vi "Export Origin - CV.vi"(8 "Error In":errorcluster, 9 "Workspace":path, 10 "Session properties":T4, 11 "CV measurement":T1={"Name"="", "Comment"="", "Time"=timestamp(0 s since 1904-01-01), "Folder"=path "", "CV properties"={"T"=0.0, "Vstart"=-0.5, "Vstop"=0.5, "Vpoints"=10.0, "Precision"=enum."Normal", "Test signal"=0.01, "Auto I range"=FALSE, "Test frequency"=100000.0, "I range"=-2.0, "V range"=10.0, "Log mapping"=FALSE, "Rel perm"=0.0, "Area"=0.0}, "GUID"=""} {"CV properties"."V range" items=["10mV"=0.01, "100mV"=0.1, "1V"=1.0, "10V"=10.0]; "CV properties"."I range" items=["100nA"=-7.0, "1µA"=-6.0, "10µA"=-5.0, "100µA"=-4.0, "1mA"=-3.0, "10mA"=-2.0]}) -> (0 "Error Out":errorcluster)   [LabVIEW 2019]
doc: "Handles export of a C-V measurement to an Origin project, displays a GUI window"
uses:
  <vilib>/Utility/sysdir.llb/System Directory Type.ctl
  Type defs/Session properties Type Def.ctl
  Type defs/CV properties Type Def.ctl
  Type defs/CV measurement Type Def.ctl
panel:
  in  "Comment":T3(array[ring])=[enum."Temperature"] caption="Parameters to be placed in comments"
  in  "Save and exit after export":bool
  in  "Export to current Origin instance":bool
  out "String":string
  in  "Path":path caption="Export file as:"
  in  "Export":bool
  in  "Cancel":bool
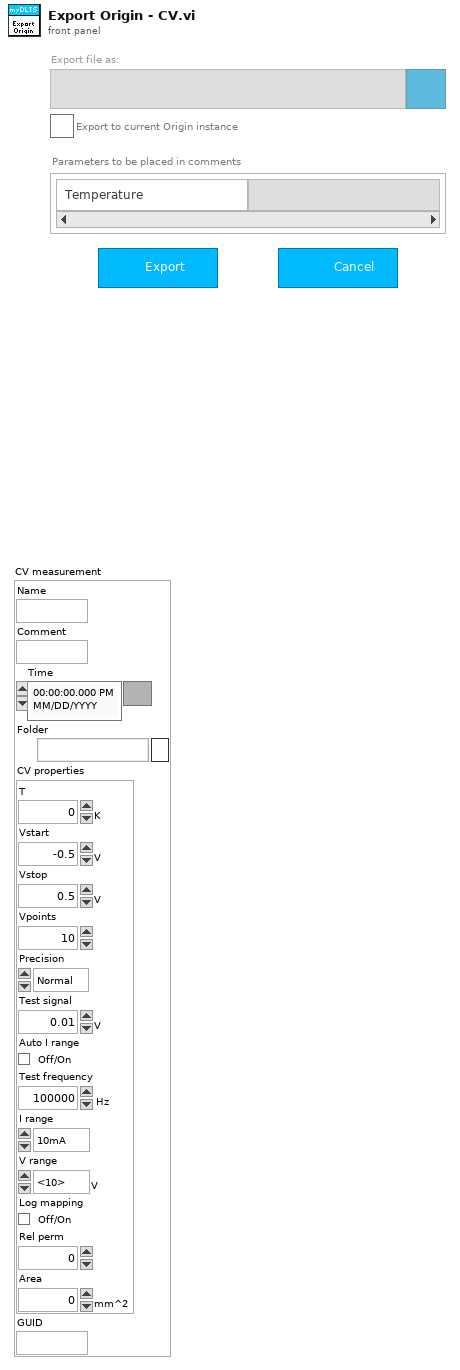
[diagram p1: front panel]
types:
  T1 = typedef "CV measurement Type Def.ctl" = cluster{"Name":string, "Comment":string, "Time":timestamp, "Folder":path, "CV properties":T2, "GUID":string}
  T2 = typedef "CV properties Type Def.ctl" = cluster{"T":dbl[unit], "Vstart":dbl[unit], "Vstop":dbl[unit], "Vpoints":dbl, "Precision":enum16{"Low (Fast)", "Normal", "High (Slow)"}, "Test signal":dbl[unit], "Auto I range":bool, "Test frequency":dbl[unit], "I range":dbl, "V range":dbl[unit], "Log mapping":bool, "Rel perm":dbl, "Area":dbl[unit]}
  T3 = enum16{"", "Temperature", "Test signal", "Test frequency", "Current range", "Voltage range"}[]
  T4 = typedef "Session properties Type Def.ctl" = cluster{"Session name":string, "Comment":string, "User":string, "Software version":dbl, "Created":timestamp, "Modified":timestamp, "Binary":bool, "GUID":string}
  T5 = enum32{"existing file", "new file", "new or existing file", "existing dir", "new dir", "new or existing dir", "existing file (use LLBs)", "new file (use LLBs)", "new or existing file (use LLBs)", "new or existing file or directory (use LLBs)", "existing dir (use LLBs)", "new dir (use LLBs)", "new or existing dir (use LLBs)", "existing file or dir", "new file or dir", "new or existing file or dir", "existing file or dir (use LLBs)", "new file or dir (use LLBs)"}
  T6 = enum8{"Enabled", "Disabled", "Disabled and Grayed Out"}
  T7 = typedef "System Directory Type.ctl" = i32
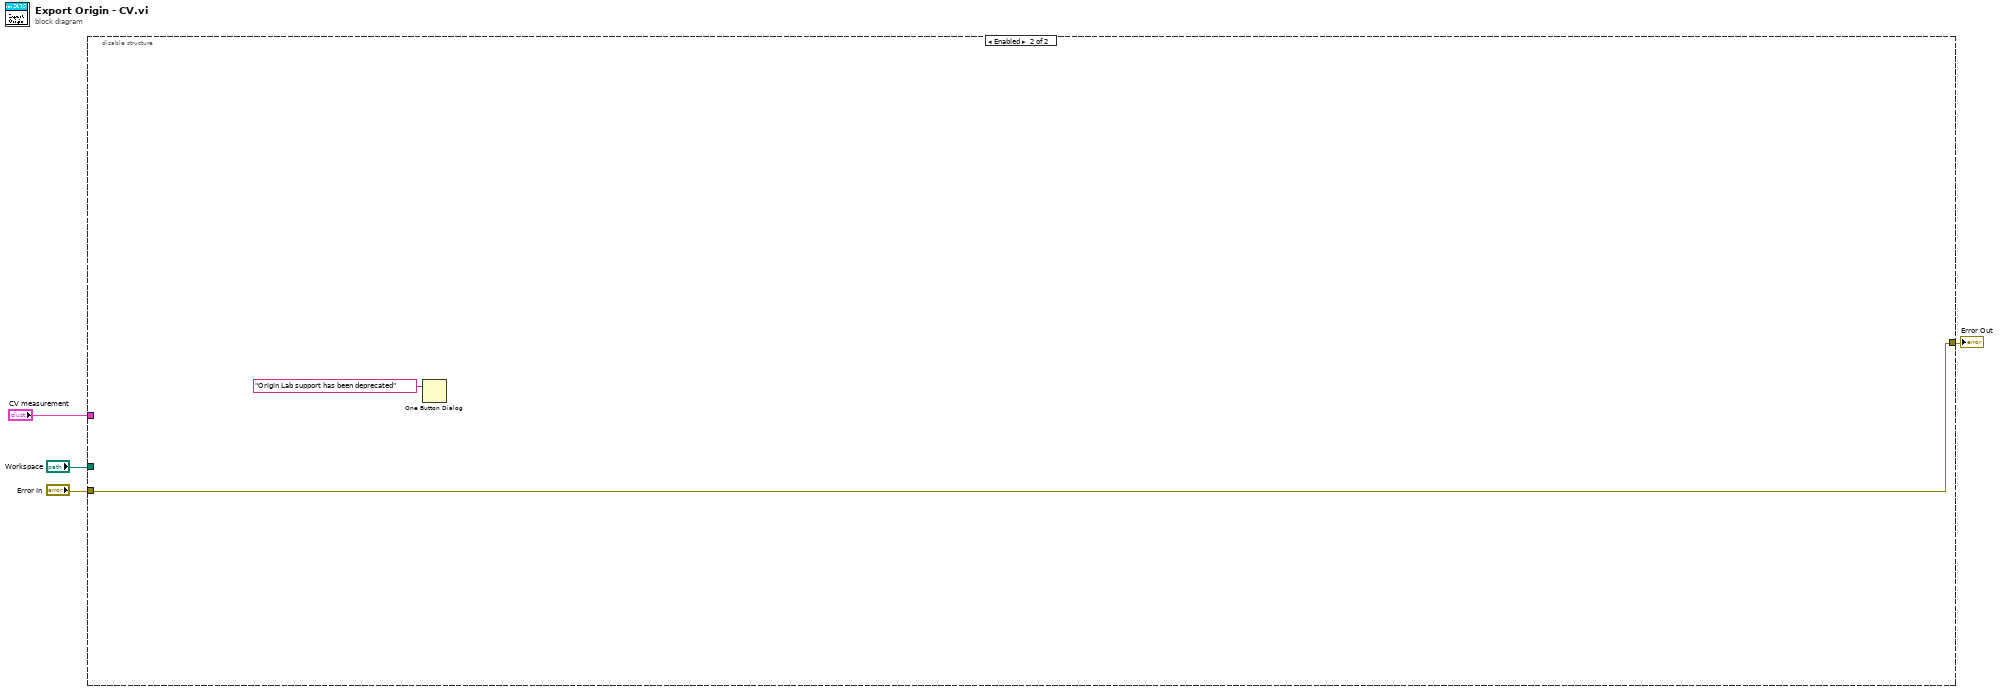
[diagram p0: block diagram]
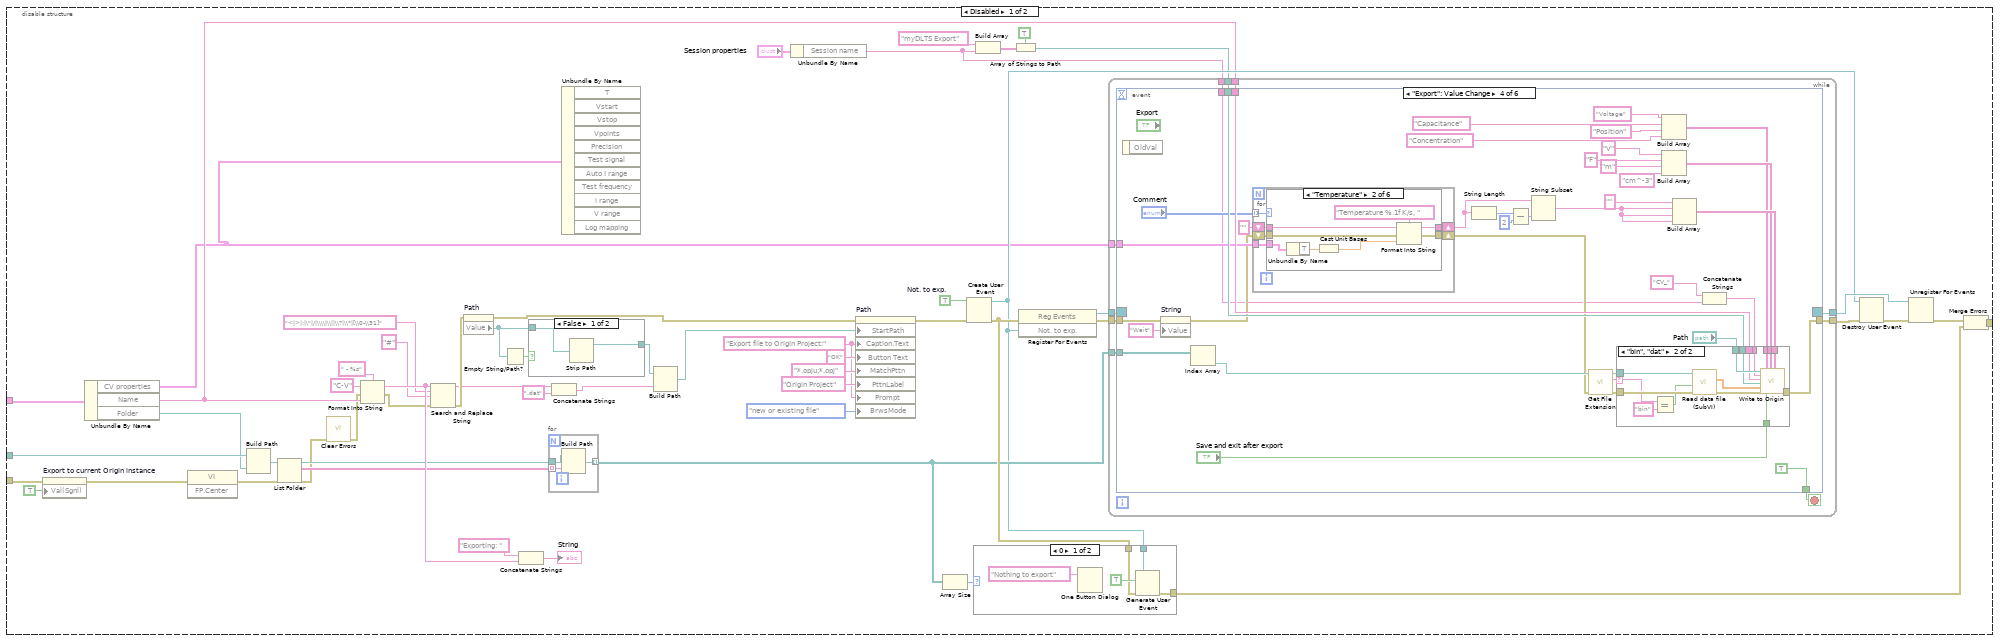
[diagram p2: hidden frame]
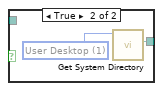
[diagram p3: hidden frame]
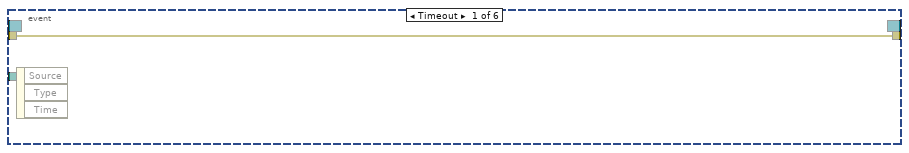
[diagram p5: hidden frame]
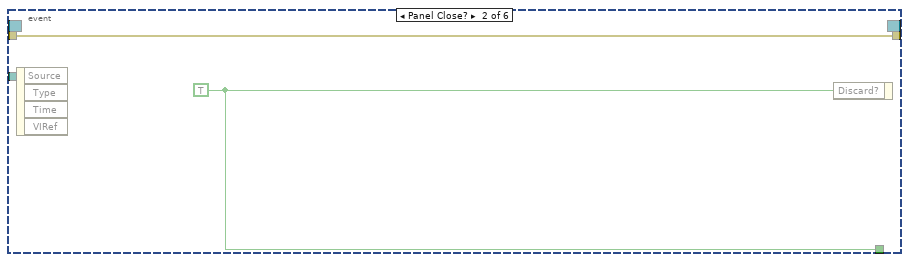
[diagram p6: hidden frame]
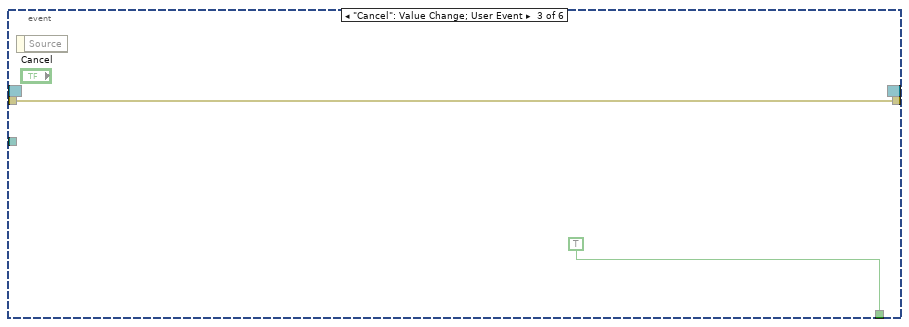
[diagram p7: hidden frame]
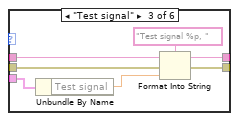
[diagram p9: hidden frame]
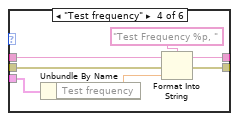
[diagram p10: hidden frame]
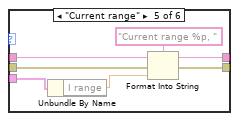
[diagram p11: hidden frame]
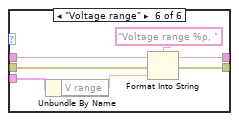
[diagram p12: hidden frame]
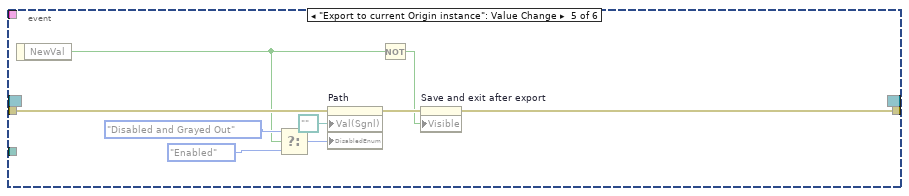
[diagram p14: hidden frame]
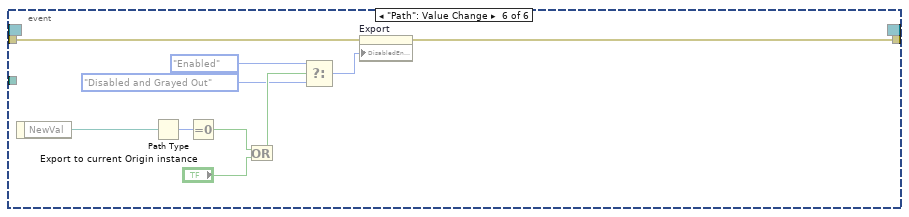
[diagram p15: hidden frame]
diagram:
  n1 = disable-structure shown="Enabled" {
    disable-tunnel: "Workspace" -> [w60 _]
    disable-tunnel: [w49 w207] -> w3
    disable-tunnel: "Error In" -> [w11 w207]
    disable-tunnel: "CV measurement" -> [w8 _]
    frame Disabled {
      w31 = "Export file to Origin Project:"
      w58 = TRUE  # Not. to exp.
      n2 = property on="Export to current Origin instance" class="Bool (strict)"(error in=w11, "Val(Sgnl)"=TRUE ("Value (Signaling)")) -> (error out=w10:errorcluster)  [unwired: 1 in, 1 out]
      n3 = Unbundle By Name(w8) -> ("CV properties"=w7:T2, "Name"=w18:string, "Folder"=w36:path)
      n4 = invoke class="VI" method="FP.Center"(error in=w10) -> (error out=w20:errorcluster)  [unwired: 2 in, 2 out]
      n5 = Build Path(base path=w60, name or relative path=w36) -> (appended path=w29:path)
      n6 = List Folder(path=w29, error in=w20) -> (path out=w28:path, filenames=w35:string[], error out=w24:errorcluster)  [unwired: 2 in, 1 out]
      n7 = call <vilib>:"Clear Errors.vi"("error in (no error)"=w24) -> ("error out"=w5:errorcluster)  [unwired: 5 in, 1 out]
      n8 = Format Into String(format string=" - %s", initial string="C-V", error in=w5, w18) -> (resulting string=w47:string, error out=w23:errorcluster)
      n9 = Search and Replace String(input string=w47, search string="<|>|:|\"|/|\\\\|\\||\\?|\\*|[\\0-\\31]", replace string="#" ("replace string (\"\")"), error in=w23) -> (result string=w22:string, error out=w25:errorcluster)  [unwired: 4 in, 2 out]
      n10 = property on="Path" class="Path"(error in=w25) -> (error out=w37:errorcluster, "Value"=w43:path)  [unwired: 1 in, 1 out]
      n11 = Empty String/Path?(string/path=w43) -> (empty?=w44:bool)
      n12 = Concatenate Strings("Exporting: " ("string"), w47) -> (→"String":string)
      n13 = case shown="False" w44 {
        tunnel: w43 -> [w65 _]
        tunnel: [w64 w66] -> w39
        frame False {
          n14 = Strip Path(path=w65) -> (stripped path=w64:path)  [unwired: 1 out]
        }
        frame True {
          w67 = T7 1 items=["User Home"=0, "User Desktop"=1, "User Documents"=2, "User Application Data"=3, "User Preferences"=4, "User Temporary"=5, "Public Documents"=6, "Public Application Data"=7, "Public Preferences"=8, "Public Cache"=13, "System Core Libraries"=9, "System Installed Libraries"=10, "Application Files"=11, "Boot Volume Root"=12] ("system directory type")
          n15 = call <vilib>:"Get System Directory.vi"("system directory type"=w67) -> ("system directory"=w66:path)  [unwired: 10 in]
        }
      }
      n16 = for {
        tunnel: w28 -> [w63]
        tunnel: [w62] -> w53 mode=indexing
        tunnel: w35 -> [w61] mode=indexing
        n17 = Build Path(base path=w63, name or relative path=w61) -> (appended path=w62:path)
      }
      n18 = Concatenate Strings(w22, ".dat" ("string")) -> (w26:string)
      n19 = Unbundle By Name(w7) -> ()  [unwired: 11 out]
      n20 = Build Path(base path=w39, name or relative path=w26) -> (appended path=w38:path)
      n21 = Unbundle By Name("Session properties") -> ("Session name"=w6:string)
      n22 = property on="Path" class="Path"(error in=w37, "StartPath"=w38, "Caption.Text"=w31, "Button Text"="OK", "MatchPttn"="*.opju;*.opj", "PttnLabel"="Origin Project", "Prompt"=w31, "BrwsMode"=T5."new or existing file" ("Browse Options:Selection Mode")) -> (error out=w55:errorcluster)  [unwired: 1 in, 1 out]
      n23 = Array Size(array=w53) -> (size(s)=w59:i32)
      n24 = Create User Event(user event datatype=w58, error in=w55) -> (user event=w19:refnum<user-event>, error out=w54:errorcluster)
      n25 = case shown="0" w59 {
        tunnel: w19 -> [w71 _]
        tunnel: w54 -> [w69 w73]
        tunnel: [w68 w73] -> w48
        frame 0 {
          n26 = One Button Dialog(message="Nothing to export") -> ()  [unwired: 1 in, 1 out]
          n27 = Generate User Event(user event=w71, event data cluster=TRUE ("event data"), error in=w69) -> (error out=w68:errorcluster)  [unwired: 1 in, 1 out]
        }
        frame Default {
        }
      }
      n28 = Build Array("myDLTS Export" ("element"), w6) -> (w14:string[])
      n29 = Array of Strings to Path(0:w14, 1:TRUE ("relative")) -> (2:w13:path)
      n30 = register-events(error in=w54, w19) -> (reference out=w56:refnum<event-registration>, error out=w57:errorcluster)  [unwired: 1 in]
      n31 = while {
        tunnel: w57 -> [w83]
        tunnel: w53 -> [w81]
        tunnel: w56 -> [w80]
        tunnel: [w79] -> w51
        tunnel: w18 -> [w78]
        tunnel: w13 -> [w77]
        tunnel: [w76] -> w12
        tunnel: w7 -> [w75]
        tunnel: w6 -> [w74]
        stop <- w82 stop-if-true
        n32 = event shown="[3] \"Export\": Value Change" {
          selector: w80 -> [_ _ _ _ _ _]
          dyn-events: [_ _ _ _ _ _] -> w79
          timeout: _ -> [_ _ _ _ _ _]
          tunnel: w83 -> [w84 w85 w87 w121 w195 w202]
          tunnel: [w84 w85 w87 w124 w188 w197] -> w76
          tunnel: [_ w86 TRUE ("Discard?") TRUE _ _] -> w82
          tunnel: w81 -> [_ _ _ w126 _ _]
          tunnel: w78 -> [_ _ _ w119 _ _]
          tunnel: w77 -> [_ _ _ w118 _ _]
          tunnel: w75 -> [_ _ _ w104 _ _]
          tunnel: w74 -> [_ _ _ w89 _ _]
          event Timeout {
            n33 = event-data() -> ()  [unwired: 1 in, 3 out]
          }
          event Panel Close? {
            w86 = TRUE ("Discard?")
            n34 = event-data() -> ()  [unwired: 1 in, 4 out]
            n35 = event-data("Discard?"=w86) -> ()  [unwired: 1 in, 1 out]
          }
          event "Cancel": Value Change; User Event {
            n36 = event-data() -> ()  [unwired: 1 in, 1 out]
          }
          event "Export": Value Change {
            n37 = event-data() -> ()  [unwired: 1 in, 1 out]
            n38 = property on="String" class="Str"(error in=w121, "Value"="Wait" ("String")) -> (error out=w103:errorcluster)  [unwired: 1 in, 1 out]
            n39 = Index Array(array=w126) -> (element=w114:path)  [unwired: 1 in]
            n40 = for {
              tunnel: "Comment" -> [w132] mode=indexing
              tunnel: w104 -> [w131]
              shift-right: [w130] -> w102
              shift-left: w103 -> [w129]
              shift-right: [w128] -> w100
              shift-left: "" -> [w127]
              n41 = case shown="\"Temperature\"" w132 {
                tunnel: w131 -> [_ w138 w143 w150 w157 w164]
                tunnel: [w133 w142 w147 w152 w161 w168] -> w130
                tunnel: w129 -> [w133 w140 w145 w154 w158 w165]
                tunnel: [w134 w141 w146 w151 w160 w167] -> w128
                tunnel: w127 -> [w134 w139 w144 w153 w159 w166]
                frame "", Default {
                }
                frame "Temperature" {
                  n42 = Unbundle By Name(w138) -> ("T"=w137:dbl[unit])
                  n43 = Cast Unit Bases(0:w137) -> (2:w135:dbl)  [unwired: 1 in]
                  n44 = Format Into String(format string="Temperature %.1f K/s, ", initial string=w139, error in=w140, w135) -> (resulting string=w141:string, error out=w142:errorcluster)
                }
                frame "Test signal" {
                  n45 = Unbundle By Name(w143) -> ("Test signal"=w148:dbl[unit])
                  n46 = Format Into String(format string="Test signal %p, ", initial string=w144, error in=w145, w148) -> (resulting string=w146:string, error out=w147:errorcluster)
                }
                frame "Test frequency" {
                  n47 = Unbundle By Name(w150) -> ("Test frequency"=w155:dbl[unit])
                  n48 = Format Into String(format string="Test Frequency %p, ", initial string=w153, error in=w154, w155) -> (resulting string=w151:string, error out=w152:errorcluster)
                }
                frame "Current range" {
                  n49 = Unbundle By Name(w157) -> ("I range"=w162:dbl)
                  n50 = Format Into String(format string="Current range %p, ", initial string=w159, error in=w158, w162) -> (resulting string=w160:string, error out=w161:errorcluster)
                }
                frame "Voltage range" {
                  n51 = Unbundle By Name(w164) -> ("V range"=w169:dbl[unit])
                  n52 = Format Into String(format string="Voltage range %p, ", initial string=w166, error in=w165, w169) -> (resulting string=w167:string, error out=w168:errorcluster)
                }
              }
            }
            n53 = String Length(string=w100) -> (length=w99:i32)
            n54 = Subtract(x=w99, y=2) -> (x-y=w98:i32)
            n55 = String Subset(string=w100, length (rest)=w98) -> (substring=w96:string)  [unwired: 1 in]
            n56 = call <vilib>:"Get File Extension.vi"("error in (no error)"=w102, "file"=w114) -> ("error out"=w116:errorcluster, "lowercase file extension"=w115:string, "dup file"=w117:path)  [unwired: 5 in, 2 out]
            n57 = Build Array("Voltage", "Capacitance", "Position" ("element"), "Concentration" ("element")) -> (w105:string[])
            n58 = Build Array("V", "F", "m" ("element"), "cm^-3" ("element")) -> (w106:string[])
            n59 = Build Array("", w96, w96, w96) -> (w107:string[])
            n60 = Concatenate Strings("CV_" ("Book name"), w89) -> (w90:string)
            n61 = case shown="\"bin\", \"dat\"" w115 {
              selector: w115 -> [_ w172]
              tunnel: w117 -> [_ w186]
              tunnel: w116 -> [w171 w185]
              tunnel: "Path" -> [_ w181]
              tunnel: w105 -> [_ w180]
              tunnel: w106 -> [_ w179]
              tunnel: w107 -> [_ w178]
              tunnel: [w171 w177] -> w124
              tunnel: "Save and exit after export" -> [_ w176]
              tunnel: w90 -> [_ w175]
              tunnel: w119 -> [_ w174]
              tunnel: w118 -> [_ w173]
              frame "False", Default {
              }
              frame "bin", "dat" {
                n62 = Equal?(x=w172, y="bin") -> (x = y?=w184:bool)
                n63 = call "Read data file (SubVI).vi"("error in"=w185, "Binary"=w184, "file path in"=w186) -> ("error out"=w182:errorcluster, "2D data"=w183:dbl[][])  [unwired: 6 in, 1 out]
                n64 = call "Write to Origin.vi"("Origin Project Path"=w181, "Book name"=w175, "Sheet name"=w174, "Folder name"=w173, "Data"=w183, "error in (no error)"=w182, "Column name"=w180, "Save and exit"=w176, "Column unit"=w179, "Column comment"=w178) -> ("error out"=w177:errorcluster)  [unwired: 9 in]
              }
            }
          }
          event "Export to current Origin instance": Value Change {
            n65 = event-data() -> ("NewVal"=w190:bool)  [unwired: 1 in]
            n66 = Select(t=T6."Disabled and Grayed Out" ("Disabled"), s=w190, f=T6."Enabled" ("Disabled")) -> (s? t:f=w191:T6)
            n67 = property on="Path" class="Path"(error in=w195, "Val(Sgnl)"=path "" ("Value (Signaling)"), "DisabledEnum"=w191) -> (error out=w194:errorcluster)  [unwired: 1 in, 1 out]
            n68 = Not(x=w190) -> (.not. x?=w189:bool)
            n69 = property on="Save and exit after export" class="Bool (strict)"(error in=w194, "Visible"=w189) -> (error out=w188:errorcluster)  [unwired: 1 in, 1 out]
          }
          event "Path": Value Change {
            n70 = event-data() -> ("NewVal"=w206:path)  [unwired: 1 in]
            n71 = Path Type(1:w206) -> (0:w205:i16)
            n72 = Equal To 0?(x=w205) -> (x = 0?=w203:bool)
            n73 = Or(x=w203, y="Export to current Origin instance") -> (x .or. y?=w201:bool)
            n74 = Select(t=T6."Enabled" ("Disabled"), s=w201, f=T6."Disabled and Grayed Out") -> (s? t:f=w200:T6)
            n75 = property on="Export" class="Bool"(error in=w202, "DisabledEnum"=w200) -> (error out=w197:errorcluster)  [unwired: 1 in, 1 out]
          }
        }
      }
      n76 = Destroy User Event(user event=w19, error in=w12) -> (error out=w52:errorcluster)
      n77 = Unregister For Events(event registration refnum=w51, error in=w52) -> (error out=w50:errorcluster)
      n78 = Merge Errors(w50, w48) -> (w49:errorcluster)
    }
    frame Enabled {
      n79 = One Button Dialog(message="Origin Lab support has been deprecated") -> ()  [unwired: 1 in, 1 out]
    }
  }
  "Error Out" <- w3
